vi "Memory Cell to phi.vi"(10 "Memory Cell":T1={"type"=enum."float", "x"=0.0, "y"=0.0, "z"=0.0, "w"=0.0}) -> (2 "float out":dbl)   [LabVIEW 2023]
uses:
  Type Definitions/Memory Cell.ctl
  Type Definitions/Memory Cell Type Enum.ctl
  Shared Components/Orient3d Class/Orient3d.lvclass
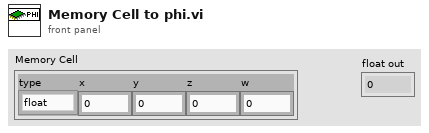
[diagram p1: front panel]
types:
  T1 = typedef "Memory Cell.ctl" = cluster{"type":T2, "x":dbl, "y":dbl, "z":dbl, "w":dbl}
  T2 = typedef "Memory Cell Type Enum.ctl" = enum16{"integer", "float", "vector", "rotation"}
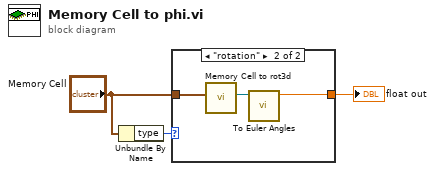
[diagram p0: block diagram]
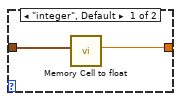
[diagram p2: hidden frame]
diagram:
  n1 = Unbundle By Name("Memory Cell") -> ("type"=w1:T2)
  n2 = case shown="\"rotation\"" w1 {
    tunnel: "Memory Cell" -> [w5 w8]
    tunnel: [w4 w6] -> w3
    frame "integer", Default {
      n3 = call "Memory Cell to float.vi"("Memory Cell"=w5) -> ("float out"=w4:dbl)  [unwired: 10 in]
    }
    frame "rotation" {
      n4 = call "Memory Cell to rot3d.vi"("Memory Cell"=w8) -> ("Orient3d out"=w7:refnum<class "Orient3d.lvclass">)  [unwired: 10 in]
      n5 = call "To Euler Angles.vi"("Orient3d in"=w7) -> ("psi/yaw"=w6:dbl)  [unwired: 7 in, 3 out]
    }
  }
  "float out" <- w3
